vi "Measure Average Power.vi"(8 "error in":errorcluster, 9 "# Samples in":dbl, 10 "Channel in":T1, 11 "2936r in":refnum<class "2936r.lvclass">) -> (0 "error out":errorcluster, 1 "# Samples out":dbl, 2 "Average Power":dbl, 3 "2936r out":refnum<class "2936r.lvclass">)   [LabVIEW 2018, in "2936r.lvlib" / "2936r.lvclass"]
uses:
  2936r.lvclass
  PPLs/Optical Power Meter/Optical Power Meter.lvlibp/Custom Controls/Channel List.ctl
  2936r.lvclass/2936r.ctl
  <vilib>/Analysis/baseanly.llb/Mean (DBL).vi
  <vilib>/Analysis/NI_AALBase.lvlib
  PPLs/Optical Power Meter/Optical Power Meter.lvlibp
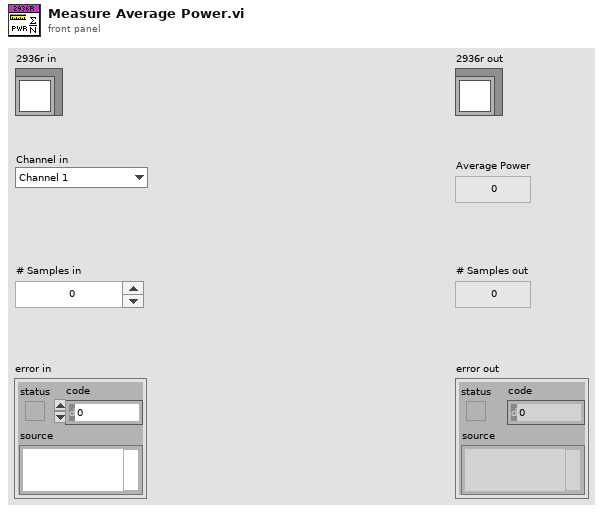
[diagram p1: front panel]
types:
  T1 = typedef "Optical Power Meter.lvlibp/Channel List.ctl" = enum16{"Channel 1", "Channel 2", "Channel 3", "Channel 4"}
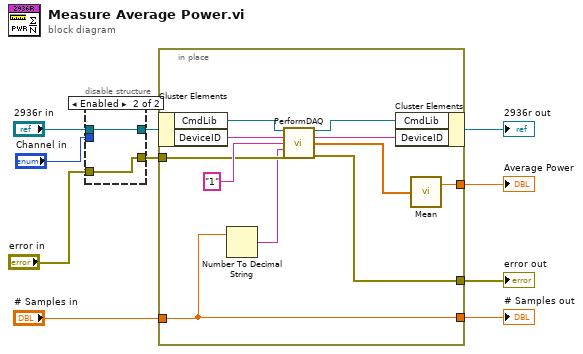
[diagram p0: block diagram]
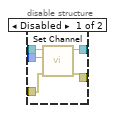
[diagram p2: hidden frame]
diagram:
  n1 = disable-structure shown="Enabled" {
    disable-tunnel: "2936r in" -> [w15 w17]
    disable-tunnel: "Channel in" -> [w14 _]
    disable-tunnel: [w13 w17] -> w3
    disable-tunnel: [w12 w16] -> w2
    disable-tunnel: "error in" -> [w11 w16]
    frame Disabled {
      n2 = call-dynamic "Set Channel.vi"("error in (no error)"=w11, "Channel"=w14, "2936r in"=w15) -> ("error out"=w12:errorcluster, "2936r out"=w13:refnum<class "2936r.lvclass">)  [unwired: 7 in]
    }
    frame Enabled {
    }
  }
  n3 = in-place {
    in-place-border: w2 -> [w23]
    in-place-border: [w22] -> w9
    in-place-border: [w20] -> w8
    in-place-border: "# Samples in" -> [w19]
    in-place-border: [w19] -> w6
    n4 = in-place-cluster #1(w3) -> ("CmdLib"=w28:refnum<k24>, "DeviceID"=w26:string)
    n5 = Number To Decimal String(number=w19) -> (decimal integer string=w18:string)  [unwired: 1 in]
    n6 = call <instrlib>:"PerformDAQ.vi"("PM Cmds In"=w28, "Device Key In"=w26, "Interval"="1", "Sample Size"=w18, "error in"=w23) -> ("PM Cmds Out"=w27:refnum<k24>, "Device Key Out"=w25:string, "Data Acquisition"=w21:dbl[], "error out"=w22:errorcluster)  [unwired: 7 in]
    n7 = in-place-cluster #1("CmdLib"=w27, "DeviceID"=w25) -> (→"2936r out":refnum<class "2936r.lvclass">)
    n8 = call-poly <vilib>:"Mean.vi"("X"=w21) -> ("mean"=w20:dbl)  [unwired: 1 out]
  }
  "error out" <- w9
  "Average Power" <- w8
  "# Samples out" <- w6
